vi "Format into String.vi"() -> ()   [LabVIEW 2016]
panel:
  in  "Boolean":bool
  in  "final string":string
  out "resulting string":string
  in  "input 1":dbl
  in  "initial string":string
  in  "format string":string
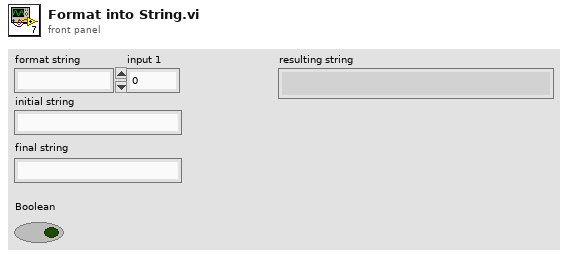
[diagram p1: front panel]
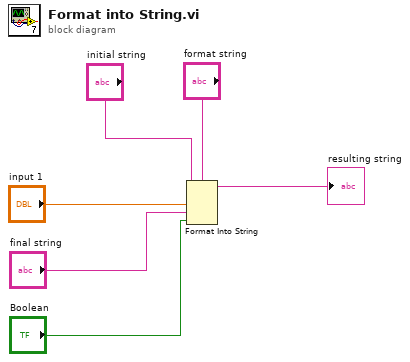
[diagram p0: block diagram]
diagram:
  n1 = Format Into String(format string="format string", initial string="initial string", "input 1", "final string", "Boolean") -> (resulting string=→"resulting string":string)  [unwired: 1 in, 1 out]
